vi "Create Table Polymorphic.vi"   [LabVIEW 2019]
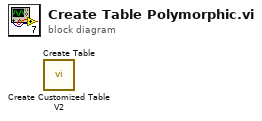
[diagram p0: block diagram]
diagram:
  n1 = call <vilib>:"Create Customized Table V2.vi"() -> ()  [unwired: 13 in, 3 out]
  n2 = call <userlib>:"Create Table.vi"() -> ()  [unwired: 13 in, 3 out]
